vi "处理TDMS文件.vi"(8 "String引用":refnum<vi>, 9 "滑动杆引用":refnum<vi>, 10 "停止引用":refnum<data-value>, 11 "文件路径数组":path[](array[path])) -> ()   [LabVIEW 2018]
panel:
  # "直接写入当前处理的文件数"
  # "直接写入当前处理的文件名"
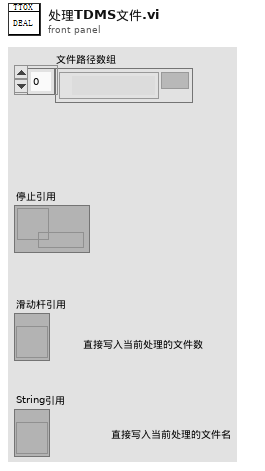
[diagram p1: front panel]
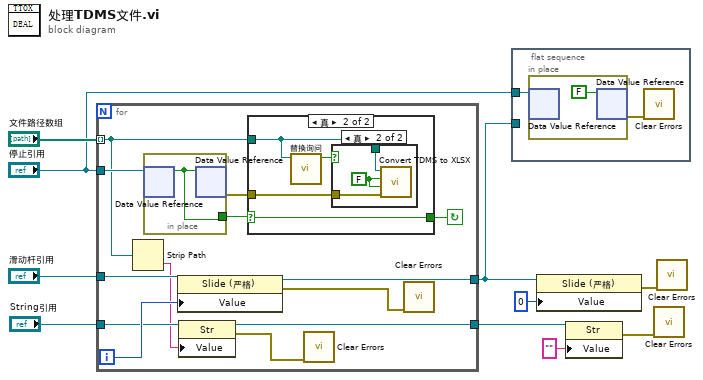
[diagram p0: block diagram]
diagram:
  n1 = for {
    tunnel: "文件路径数组" -> [w14] mode=indexing
    tunnel: "停止引用" -> [w23]
    tunnel: "滑动杆引用" -> [w17]
    tunnel: [w16] -> w5
    tunnel: "String引用" -> [w15]
    tunnel: [w11] -> w3
    i -> [w19]
    stop <- w20 continue-if-true
    n2 = Strip Path(path=w14) -> (name=w13:string)  [unwired: 1 out]
    n3 = in-place {
      in-place-border: [w32] -> w21
      n4 = in-place-dvr #1(w23) -> (w32:bool)  [unwired: 1 out]
      n5 = in-place-dvr #1(w32) -> (w22:errorcluster)  [unwired: 1 out]
    }
    n6 = property class="Slide (严格)"(reference=w17, "Value"=w19) -> (reference out=w16:refnum<vi>, error out=w18:errorcluster)  [unwired: 1 in]
    n7 = property class="Str"(reference=w15, "Value"=w13) -> (reference out=w11:refnum<vi>, error out=w12:errorcluster)  [unwired: 1 in]
    n8 = case shown="真" w21 {
      selector: w21 -> [w24 w28]
      tunnel: w14 -> [_ w27]
      tunnel: w22 -> [_ w25]
      tunnel: [w24 w28] -> w20
      frame False {
      }
      frame True {
        n9 = call "替换询问.vi"("TDMS/TDM File"=w27) -> ("替换"=w26:bool)  [unwired: 10 in]
        n10 = case shown="真" w26 {
          tunnel: w27 -> [_ w30]
          tunnel: w25 -> [_ w29]
          frame False {
          }
          frame True {
            w31 = FALSE ("Remove Extra Properties? (T)")
            n11 = call "Convert TDMS to XLSX.vi"("error in"=w29, "Show Configure Dialog?"=w31, "Remove Extra Properties? (T)"=w31, "Path to TDMS/TDM File"=w30) -> ()  [unwired: 7 in, 1 out]
          }
        }
      }
    }
    n12 = call <vilib>:"Clear Errors.vi"("error in (no error)"=w12) -> ()  [unwired: 5 in, 2 out]
    n13 = call <vilib>:"Clear Errors.vi"("error in (no error)"=w18) -> ()  [unwired: 5 in, 2 out]
  }
  n14 = flat-sequence {
    tunnel: "停止引用" -> [w34]
    tunnel: w5 -> [_]
    frame #0 {
      n15 = in-place {
        n16 = in-place-dvr #2(w34) -> ()  [unwired: 2 out]
        n17 = in-place-dvr #2(FALSE ("数据值")) -> (w33:errorcluster)  [unwired: 1 out]
      }
      n18 = call <vilib>:"Clear Errors.vi"("error in (no error)"=w33) -> ()  [unwired: 5 in, 2 out]
    }
  }
  n19 = property class="Slide (严格)"(reference=w5, "Value"=u8 0 ("值")) -> (error out=w7:errorcluster)  [unwired: 1 in, 1 out]
  n20 = property class="Str"(reference=w3, "Value"="" ("值")) -> (error out=w1:errorcluster)  [unwired: 1 in, 1 out]
  n21 = call <vilib>:"Clear Errors.vi"("error in (no error)"=w1) -> ()  [unwired: 5 in, 2 out]
  n22 = call <vilib>:"Clear Errors.vi"("error in (no error)"=w7) -> ()  [unwired: 5 in, 2 out]
